vi "Get Plugin OS from Project Name.vi"(3 "Project Path":path) -> (1 "Plugin OS":T1=enum."Env Server" caption="OS")   [LabVIEW 2023, in "Plugin Generator.lvlib"]
uses:
  Plugin Generator.lvlib
  Typedef/Plugin OS.ctl
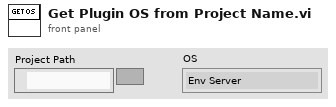
[diagram p1: front panel]
types:
  T1 = typedef "Plugin Generator.lvlib/Plugin OS.ctl" = enum16{"Linux RT", "Env Server"}
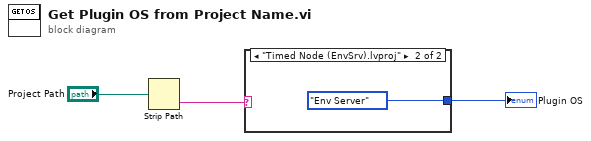
[diagram p0: block diagram]
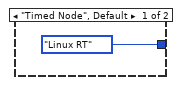
[diagram p2: hidden frame]
diagram:
  n1 = Strip Path(path="Project Path") -> (name=w2:string)  [unwired: 1 out]
  n2 = case shown="\"Timed Node (EnvSrv).lvproj\"" w2 {
    tunnel: [Plugin_OS."Linux RT" ("Plugin OS") Plugin_OS."Env Server" ("Plugin OS")] -> w1
    frame "Timed Node", Default {
    }
    frame "Timed Node (EnvSrv).lvproj" {
    }
  }
  "Plugin OS" <- w1
